vi "Set EnFlo Tunnel inlet Fans.vi"(1 "Tunnel Velocity m/s":dbl) -> (0 "Error Message":string)   [LabVIEW 2022 SP3]
uses:
  Anemometry/Anemometry Sub Vis/Globals/Constants_global.vi
panel:
  out "Channel Values":dbl[](array[numeric])
  out "Channel Names":string[](array[string])
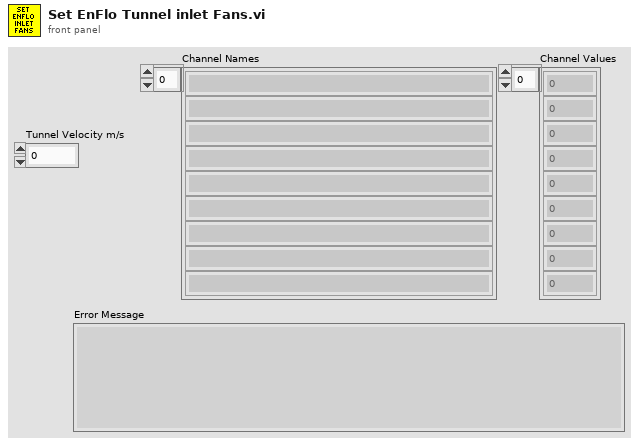
[diagram p1: front panel]
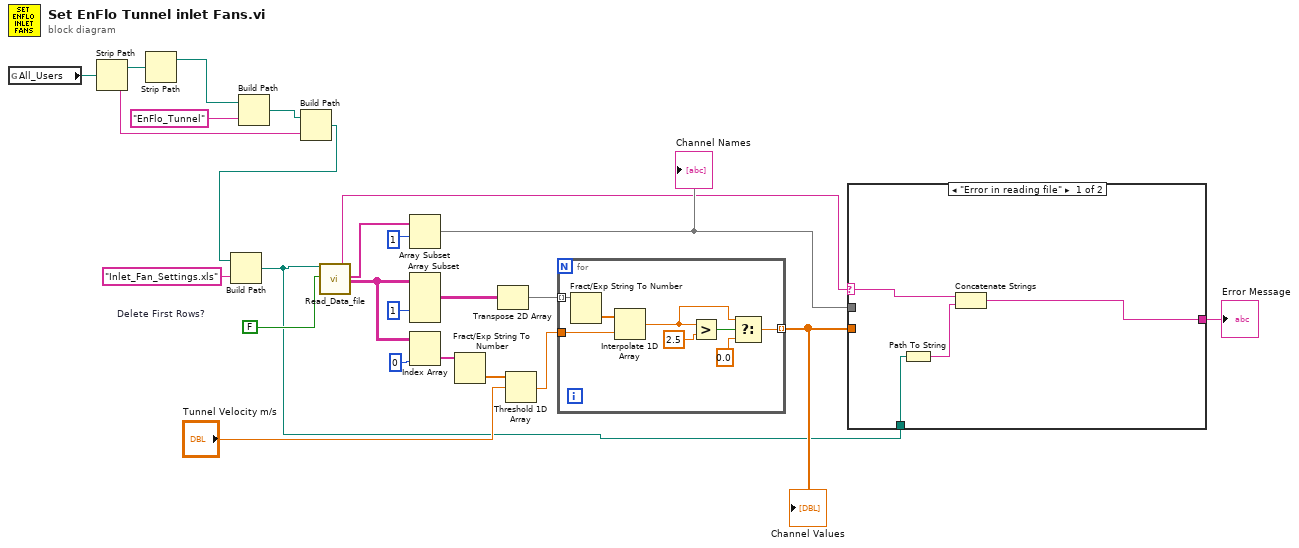
[diagram p0: block diagram]
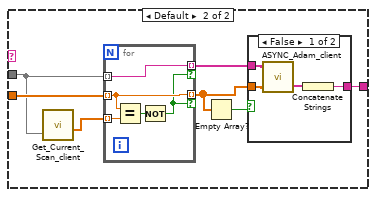
[diagram p2: hidden frame]
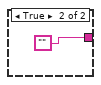
[diagram p3: hidden frame]
diagram:
  w25 = FALSE  # Delete First Rows?
  n1 = global read "Constants_global.vi" "All_Users"() -> (w7:path)
  n2 = Strip Path(path=w7) -> (stripped path=w6:path, name=w2:string)
  n3 = Strip Path(path=w6) -> (stripped path=w5:path)  [unwired: 1 out]
  n4 = Build Path(base path=w5, name or relative path="EnFlo_Tunnel") -> (appended path=w3:path)
  n5 = Build Path(base path=w3, name or relative path=w2) -> (appended path=w1:path)
  n6 = Build Path(base path=w1, name or relative path="Inlet_Fan_Settings.xls") -> (appended path=w9:path)
  n7 = call "Read_Data_file.vi"("Results file"=w9, "Delete First Rows?"=w25) -> ("Filetype"=w10:string, "Ch names Out"=w13:string[], "Channel Values Out"=w17:string[][])  [unwired: 8 in, 7 out]
  n8 = Array Subset(array=w13, index=1) -> (w23:string[])  [unwired: 1 in]
  "Channel Names" <- w23
  n9 = Array Subset(array=w17, index (col)=1 ("index")) -> (w20:string[][])  [unwired: 3 in]
  n10 = Index Array(array=w17, index (col)=0 ("index (row)")) -> (element=w15:string[])  [unwired: 1 in]
  n11 = Fract/Exp String To Number(string=w15) -> (number=w14:dbl[])  [unwired: 3 in, 1 out]
  n12 = Transpose 2D Array(2D array=w20) -> (transposed array=w21:string[][])
  n13 = Threshold 1D Array(2:"Tunnel Velocity m/s", 3:w14) -> (0:w11:dbl)  [unwired: 1 in]
  n14 = for {
    tunnel: w21 -> [w33] mode=indexing
    tunnel: w11 -> [w32]
    tunnel: [w26] -> w22 mode=indexing
    n15 = Fract/Exp String To Number(string=w33) -> (number=w31:dbl[])  [unwired: 3 in, 1 out]
    n16 = Interpolate 1D Array(1:w32, 2:w31) -> (0:w28:dbl)
    n17 = Greater?(x=w28, y=2.5) -> (0:w29:bool)
    n18 = Select(t=w28, s=w29, f=0.0) -> (s? t:f=w26:dbl)
  }
  "Channel Values" <- w22
  n19 = case shown="\"Error in reading file\"" w10 {
    selector: w10 -> [w37 _]
    tunnel: w22 -> [_ w43]
    tunnel: w23 -> [_ w40]
    tunnel: w9 -> [w35 _]
    tunnel: [w34 w42] -> w8
    frame "Error in reading file" {
      n20 = Path To String(path=w35) -> (string=w36:string)
      n21 = Concatenate Strings(w37, w36) -> (w34:string)
    }
    frame Default {
      n22 = call "Get_Current_Scan_client.vi"("multipleChannels"=w40) -> ("Numerical Values"=w44:dbl[])  [unwired: 1 in, 3 out]
      n23 = for {
        tunnel: w44 -> [w49] mode=indexing
        tunnel: w43 -> [w46] mode=indexing
        tunnel: [w47] -> w41 mode=indexing if=w45
        tunnel: w40 -> [w47] mode=indexing
        tunnel: [w46] -> w38 mode=indexing if=w45
        n24 = Equal?(x=w46, y=w49) -> (x = y?=w48:bool)
        n25 = Not(x=w48) -> (.not. x?=w45:bool)
      }
      n26 = Empty Array?(array=w38) -> (empty?=w39:bool)
      n27 = case shown="False" w39 {
        tunnel: w41 -> [w53 _]
        tunnel: w38 -> [w52 _]
        tunnel: [w50 ""] -> w42
        frame False {
          n28 = call "ASYNC_Adam_client.vi"("Values"=w52, "Channel Names"=w53) -> ("Scan Comments"=w51:string[])  [unwired: 1 in, 1 out]
          n29 = Concatenate Strings(w51) -> (w50:string)
        }
        frame True {
        }
      }
    }
  }
  "Error Message" <- w8
